vi "Display Image Features.vi"(6 "Local Data":T1, 7 "UI References":T8, 8 "error in (no error)":errorcluster, 10 "Features":string[][](array[string])) -> (0 "error out":errorcluster)   [LabVIEW 2024]
uses:
  Controls/RVHR - UI Refs.ctl
  Controls/RVHR - Local Data.ctl
  Controls/Test Cluster.ctl
  Controls/Excluded Information.ctl
  Controls/Language.ctl
  Controls/Device_Type.ctl
  <vilib>/Utility/miscctls.llb/LVRectTypeDef.ctl
  <vilib>/Utility/miscctls.llb/LVBoundsTypeDef.ctl
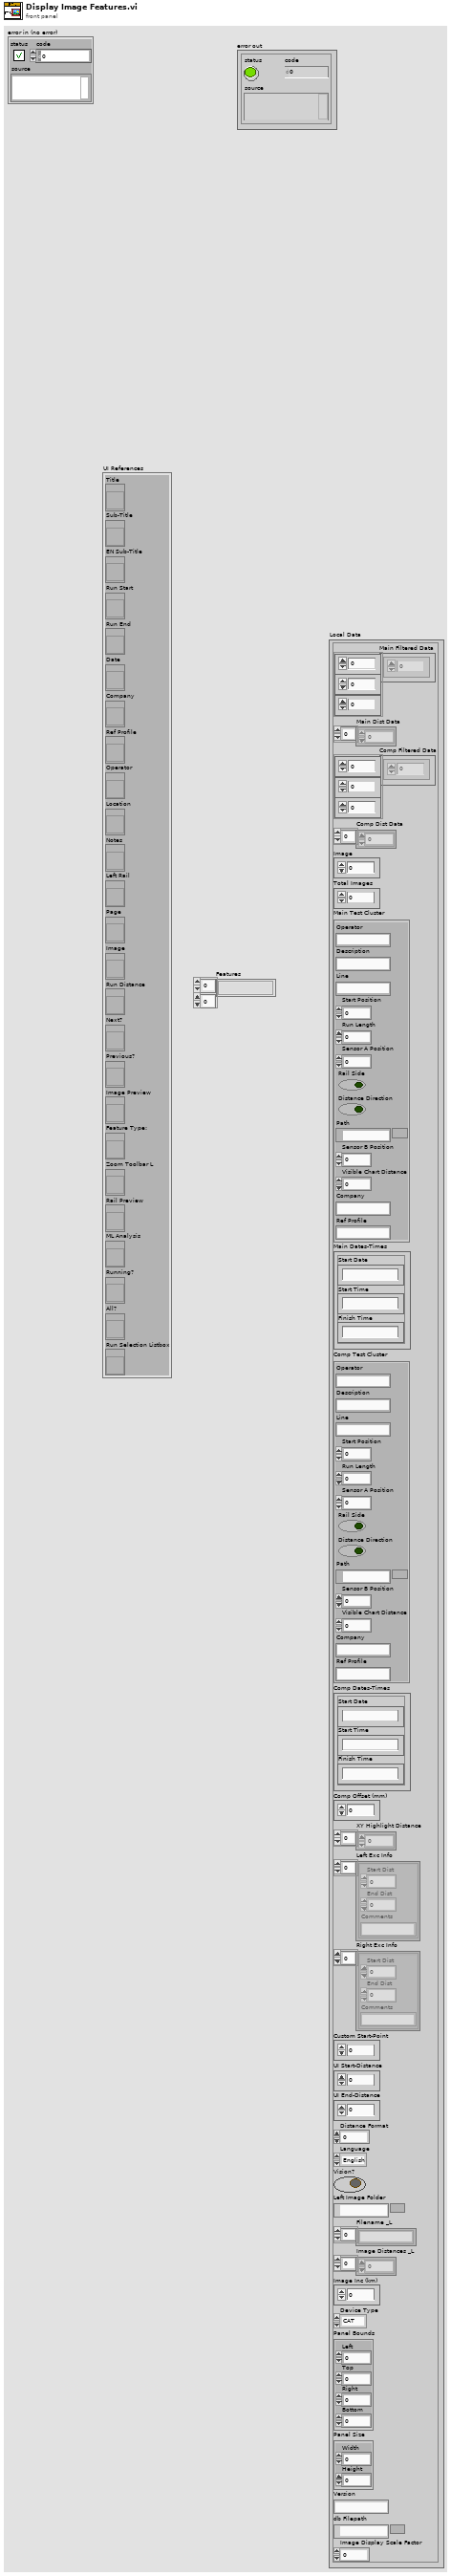
[diagram p1: front panel]
types:
  T1 = typedef "RVHR - Local Data.ctl" = cluster{"Main Filtered Data":dbl[][][], "Main Dist Data":dbl[], "Comp Filtered Data":dbl[][][], "Comp Dist Data":dbl[], "Image":u16, "Total Images":u16, "Main Test Cluster":T2, "Main Dates-Times":cluster{"Start Date":string, "Start Time":string, "Finish Time":string}, "Comp Test Cluster":T2, "Comp Dates-Times":cluster{"Start Date":string, "Start Time":string, "Finish Time":string}, "Comp Offset (mm)":i64, "XY Highlight Distance":dbl[], "Left Exc Info":T3[], "Right Exc Info":T3[], "Custom Start-Point":dbl, "UI Start-Distance":dbl, "UI End-Distance":dbl, "Distance Format":u8, "Language":T4, "Vision?":bool, "Left Image Folder":path, "Filename _L":string[], "Image Distances _L":dbl[], "Image Inc (km)":dbl, "Device Type":T5, "Panel Bounds":T6, "Panel Size":T7, "Version":string, "db Filepath":path, "Image Display Scale Factor":dbl}
  T2 = typedef "Test Cluster.ctl" = cluster{"Operator":string, "Description":string, "Line":string, "Start Position":dbl, "Run Length":dbl, "Sensor A Position":dbl, "Rail Side":bool, "Distance Direction":bool, "Path":path, "Sensor B Position":dbl, "Visible Chart Distance":dbl, "Company":string, "Ref Profile":string}
  T3 = typedef "Excluded Information.ctl" = cluster{"Start Dist":dbl, "End Dist":dbl, "Comments":string}
  T4 = typedef "Language.ctl" = enum16{"English", "Chinese", "German"}
  T5 = typedef "Device_Type.ctl" = enum16{"CAT", "Bi-CAT", "YRCA", "RCA", "RV-HR", "TV-HR"}
  T6 = typedef "LVRectTypeDef.ctl" = cluster{"Left":i16, "Top":i16, "Right":i16, "Bottom":i16}
  T7 = typedef "LVBoundsTypeDef.ctl" = cluster{"Width":u32, "Height":u32}
  T8 = typedef "RVHR - UI Refs.ctl" = cluster{"Title":refnum<vi>, "Sub-Title":refnum<vi>, "EN Sub-Title":refnum<vi>, "Run Start":refnum<vi>, "Run End":refnum<vi>, "Date":refnum<vi>, "Company":refnum<vi>, "Ref Profile":refnum<vi>, "Operator":refnum<vi>, "Location":refnum<vi>, "Notes":refnum<vi>, "Left Rail":refnum<vi>, "Page":refnum<vi>, "Image":refnum<vi>, "Run Distance":refnum<vi>, "Next?":refnum<vi>, "Previous?":refnum<vi>, "Image Preview":refnum<vi>, "Feature Type:":refnum<vi>, "Zoom Toolbar L":refnum<vi>, "Rail Preview":refnum<vi>, "ML Analysis":refnum<vi>, "Running?":refnum<vi>, "All?":refnum<vi>, "Run Selection Listbox":refnum<vi>}
  T9 = cluster{"Width":i16, "Style":enum32{"Solid", "Dash", "Dot", "DashDot", "DashDotDot"}}
  T10 = cluster{"horizontal":enum16{"left", "center", "right"}, "vertical":enum16{"top", "center", "bottom"}}
  T11 = cluster{"[0]":i32, "[1]":i32, "[2]":i32, "[3]":i32}
  T12 = enum16{"User-specified Font", "Application Font", "System Font", "Dialog Font"}
  T13 = cluster{"Font Name:":string, "Size":i16, "Strikeout?":bool, "Italic?":bool, "Underline?":bool, "Outline?":bool, "Shadow?":bool, "Bold?":bool}
  T14 = cluster{"left":i16, "top":i16, "right":i16, "bottom":i16}
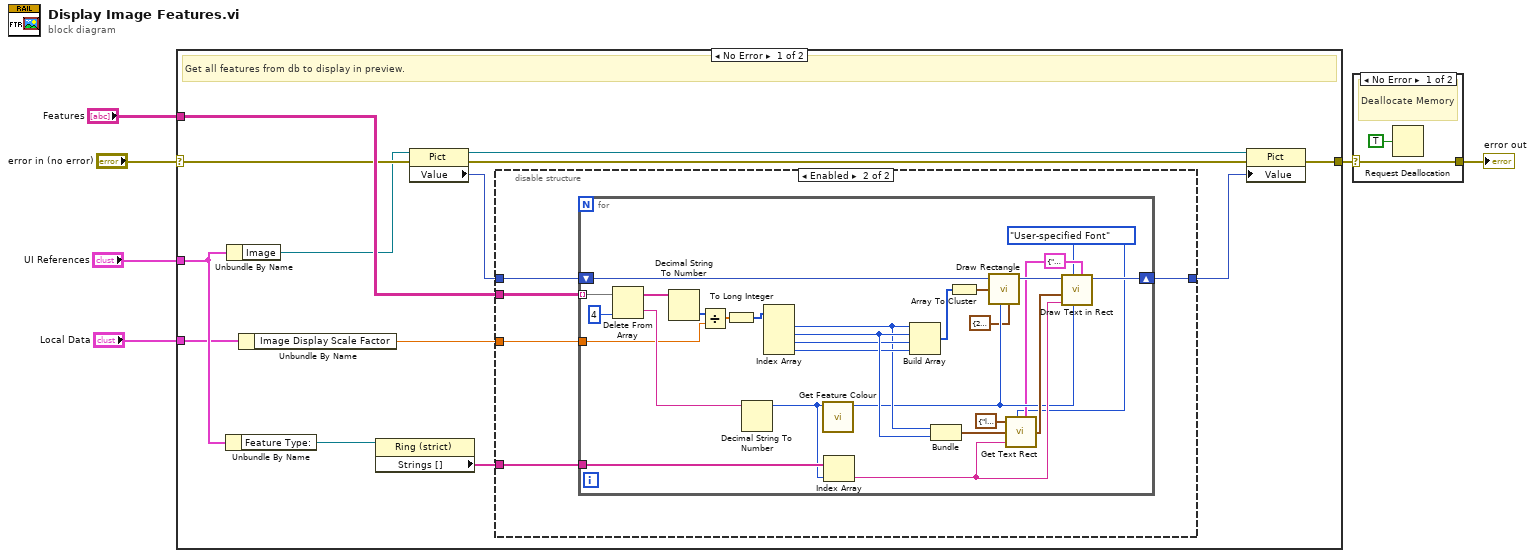
[diagram p0: block diagram]
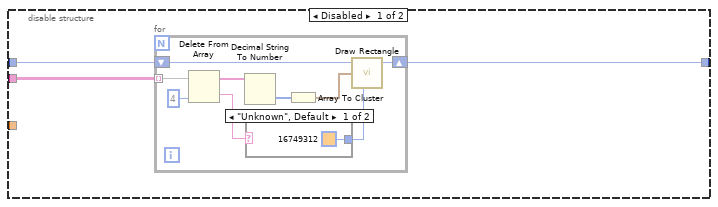
[diagram p3: hidden frame]
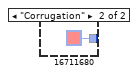
[diagram p4: hidden frame]
diagram:
  n1 = case shown="No Error" "error in (no error)" {
    selector: "error in (no error)" -> [w18 w66]
    tunnel: [w13 w66] -> w1
    tunnel: "UI References" -> [w12 _]
    tunnel: "Features" -> [w19 _]
    tunnel: "Local Data" -> [w8 _]
    frame No Error {
      # "Get all features from db to display in preview."
      n2 = Unbundle By Name(w12) -> ("Feature Type:"=w11:refnum<vi>)
      n3 = Unbundle By Name(w12) -> ("Image"=w9:refnum<vi>)
      n4 = Unbundle By Name(w8) -> ("Image Display Scale Factor"=w7:dbl)
      n5 = property class="Ring (strict)"(reference=w11) -> ("Strings []"=w10:string[])  [unwired: 1 in, 2 out]
      n6 = property class="Pict"(reference=w9, error in=w18) -> (reference out=w17:refnum<vi>, error out=w15:errorcluster, "Value"=w14:picture)
      n7 = disable-structure shown="Enabled" {
        disable-tunnel: w19 -> [w22 w38]
        disable-tunnel: [w21 w37] -> w16
        disable-tunnel: w14 -> [w20 w36]
        disable-tunnel: w10 -> [_ w35]
        disable-tunnel: w7 -> [_ w34]
        frame Disabled {
          n8 = for {
            tunnel: w22 -> [w31] mode=indexing
            shift-right: [w25] -> w21
            shift-left: w20 -> [w26]
            n9 = Delete From Array(array=w31, index=4) -> (deleted portion=w24:string, array with subset deleted=w29:string[])  [unwired: 1 in]
            n10 = Decimal String To Number(string=w29) -> (number=w28:i32[])  [unwired: 2 in, 1 out]
            n11 = case shown="\"Unknown\", Default" w24 {
              tunnel: [u32 16749312 ("color(black)") u32 16711680 ("color(black)")] -> w23
              frame "Unknown", Default {
              }
              frame "Corrugation" {
              }
            }
            n12 = Array To Cluster(array=w28) -> (cluster=w27:T11)
            n13 = call <vilib>:"Draw Rectangle.vi"("picture"=w26, "rect"=w27, "color(black)"=w23) -> ("new picture"=w25:picture)  [unwired: 6 in]
          }
        }
        frame Enabled {
          n14 = for {
            tunnel: w38 -> [w65] mode=indexing
            shift-right: [w54] -> w37
            shift-left: w36 -> [w61]
            tunnel: w35 -> [w53]
            tunnel: w34 -> [w42]
            w44 = T12."User-specified Font" ("desired font(Application)")
            w45 = T13 {"Font Name:"="Arial", "Size"=18, "Strikeout?"=FALSE, "Italic?"=FALSE, "Underline?"=FALSE, "Outline?"=FALSE, "Shadow?"=FALSE, "Bold?"=FALSE} ("[user-specified font]")
            n15 = Delete From Array(array=w65, index=4) -> (deleted portion=w55:string, array with subset deleted=w63:string[])  [unwired: 1 in]
            n16 = Decimal String To Number(string=w63) -> (number=w43:i32[])  [unwired: 2 in, 1 out]
            n17 = Divide(x=w43, y=w42) -> (x/y=w40:dbl[])
            n18 = To Long Integer(number=w40) -> (32bit integer=w41:i32[])
            n19 = Decimal String To Number(string=w55) -> (number=w52:i32)  [unwired: 2 in, 1 out]
            n20 = Index Array(array=w41) -> (element #1=w51:i32, element #2=w59:i32, element #3=w57:i32, element #4=w58:i32)  [unwired: 4 in]
            n21 = call "Get Feature Colour.vi"("Feature Type"=w52) -> ("color"=w47:u32)  [unwired: 10 in]
            n22 = Index Array(array=w53, index=w52) -> (element=w48:string)
            n23 = Build Array(w51, w59, w57, w58) -> (w56:i32[])
            n24 = Bundle(w51, w59) -> (w50:cluster{i32, i32})  [unwired: 1 in]
            n25 = Array To Cluster(array=w56) -> (cluster=w62:T11)
            n26 = call <vilib>:"Draw Rectangle.vi"("picture"=w61, "rect"=w62, "color(black)"=w47, "pen"=T9 {"Width"=2, "Style"=enum."Solid"}) -> ("new picture"=w60:picture)  [unwired: 5 in]
            n27 = call <vilib>:"Get Text Rect.vi"("alignment(left, top)"=T10 {"horizontal"=enum."left", "vertical"=enum."bottom"}, "desired font(Application)"=w44, "origin(0,0)"=w50, "text"=w48, "[user-specified font]"=w45) -> ("rect"=w49:T14)  [unwired: 4 in]
            n28 = call <vilib>:"Draw Text in Rect.vi"("[user-specified font]"=w45, "text color(black)"=w47, "desired font(Application)"=w44, "text"=w48, "rect"=w49, "picture"=w60) -> ("new picture"=w54:picture)  [unwired: 5 in]
          }
        }
      }
      n29 = property class="Pict"(reference=w17, error in=w15, "Value"=w16) -> (error out=w13:errorcluster)  [unwired: 1 out]
    }
    frame Error {
    }
  }
  n30 = case shown="No Error" w1 {
    selector: w1 -> [w67 w69]
    tunnel: [w67 w69] -> w2
    frame No Error {
      # "Deallocate Memory"
      n31 = Request Deallocation(TRUE ("flag")) -> ()
    }
    frame Error {
    }
  }
  "error out" <- w2
